vi "Results Status Update Process.vi"(8 "error in (no error)":errorcluster, 10 "TestStatusEvents":T2, 11 "TestRunner_UI_Refs":T1) -> (0 "error out":errorcluster)   [LabVIEW 2011, in "GraphicalTestRunner.lvlib"]
uses:
  GraphicalTestRunner.lvlib
  Classes/TestResult/resultStatus--enum.ctl
  Classes/TestSuite/suiteStatusChanged--Cluster.ctl
  Classes/TestSuite/suiteStatus--enum.ctl
  Classes/TestResult/TestResult.lvclass
  Classes/TestSuite/TestSuite.lvclass
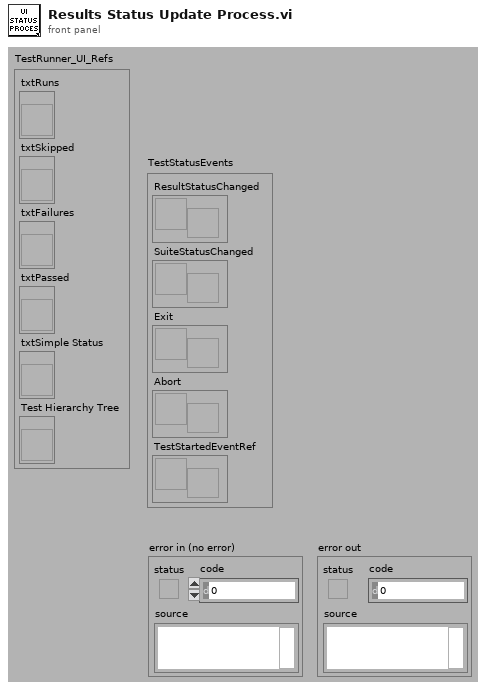
[diagram p1: front panel]
types:
  T1 = cluster{"txtRuns":refnum<vi>, "txtSkipped":refnum<vi>, "txtFailures":refnum<vi>, "txtPassed":refnum<vi>, "txtSimple Status":refnum<vi>, "Test Hierarchy Tree":refnum<vi>}
  T2 = cluster{"ResultStatusChanged":refnum<user-event>, "SuiteStatusChanged":refnum<user-event>, "Exit":refnum<user-event>, "Abort":refnum<user-event>, "TestStartedEventRef":refnum<user-event>}
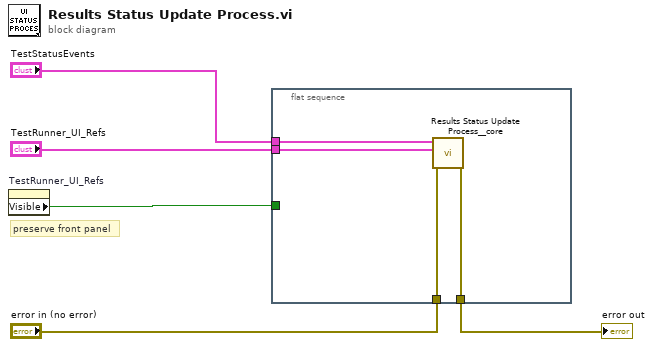
[diagram p0: block diagram]
diagram:
  # "preserve front panel"
  n1 = property on="TestRunner_UI_Refs" class="Clust (strict)"() -> ("Visible"=w1:bool)  [unwired: 2 in, 2 out]
  n2 = flat-sequence {
    tunnel: "TestStatusEvents" -> [w9]
    tunnel: "error in (no error)" -> [w8]
    tunnel: [w7] -> w3
    tunnel: "TestRunner_UI_Refs" -> [w6]
    tunnel: w1 -> [_]
    frame #0 {
      n3 = call "Results Status Update Process__core.vi"("error in (no error)"=w8, "TestRunner_UI_Refs"=w6, "TestStatusEvents"=w9) -> ("error out"=w7:errorcluster)  [unwired: 8 in]
    }
  }
  "error out" <- w3
